vi "Driving.vi"(11 "Output Cluster in":T1) -> ()   [LabVIEW 2015]
uses:
  Joytsick/Controls to Cmmnds Output Clust.ctl
  Global Vars.vi
  <vilib>/Rock Robotics/WPI/Utilities/WPI_GetSetVariantRefNum.vi
  <vilib>/Rock Robotics/WPI/RobotDrive/WPI_RobotDriveMecanumDrive_Cartesian.vi
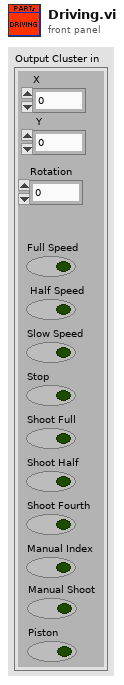
[diagram p1: front panel]
types:
  T1 = typedef "Controls to Cmmnds Output Clust.ctl" = cluster{"X ":dbl, " Y":dbl, "Rotation":dbl, "Full Speed":bool, " Half Speed":bool, "Slow Speed":bool, "Stop":bool, "Shoot Full":bool, "Shoot Half":bool, "Shoot Fourth":bool, "Manual Index":bool, "Piston":bool, "Manual Shoot":bool}
  T2 = typedef "WPI_RobotDriveDevRef.ctl" = cluster{"DevStatus":errorcluster, "Motors[]":T3[], "Square Inputs":bool, "Max Output":dbl}
  T3 = typedef "WPI_MotorControlDeviceRef.ctl" = cluster{"DeviceStatus":errorcluster, "Type":T4, "PWM":cluster{"PWM Channel":T5, "DeadBand":T6}, "CAN":cluster{"Device Number":u8, "Control Mode":T7, "Semaphore":T8, "Max Vout":dbl, "TalonSRX Control Mode":T9}, "Invert":bool}
  T4 = typedef "WPI_MotorControlType.ctl" = enum16{"PWM", "CAN", "CANTalonSRX"}
  T5 = typedef "FPGA_DIOPWMChannel.ctl" = enum8{"PWM 0", "PWM 1", "PWM 2", "PWM 3", "PWM 4", "PWM 5", "PWM 6", "PWM 7", "PWM 8", "PWM 9", "PWM MXP 0", "PWM MXP 1", "PWM MXP 2", "PWM MXP 3", "PWM MXP 4", "PWM MXP 5", "PWM MXP 6", "PWM MXP 7", "PWM MXP 8", "PWM MXP 9", "Invalid"}
  T6 = typedef "WPI_PWMDeadband.ctl" = cluster{"Name":string, "maxPositivePwm":i32, "minPositivePwm":i32, "centerPwm":i32, "maxNegativePwm":i32, "minNegativePwm":i32, "angularRange":u16}
  T7 = typedef "WPI_CANJaguar_ControlMode.ctl" = enum8{"Percent VBus", "Current", "Speed", "Position", "Voltage"}
  T8 = typedef "Semaphore RefNum" = refnum<k1>
  T9 = typedef "WPI_CANTalonSRX_APIControlMode.ctl" = enum8{"Percent VBus", "Speed", "Position", "Slave", "Unchanged / Invalid", "Voltage Compensation", "Current", "Motion Profile"}
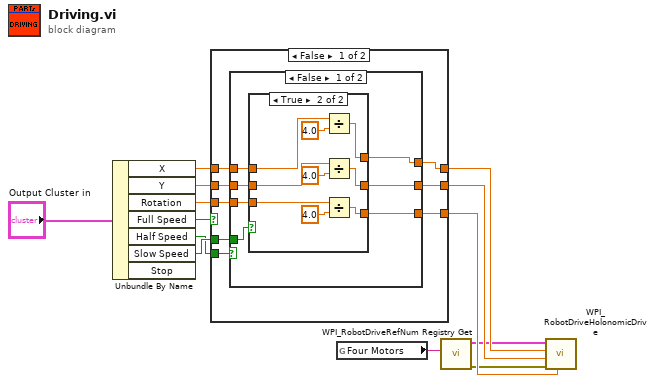
[diagram p0: block diagram]
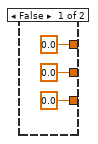
[diagram p2: hidden frame]
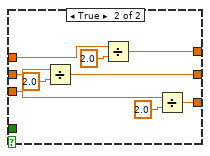
[diagram p3: hidden frame]
diagram:
  n1 = Unbundle By Name("Output Cluster in") -> ("X"=w7:dbl, "Y"=w8:dbl, "Rotation"=w10:dbl, "Full Speed"=w5:bool, "Half Speed"=w12:bool, "Slow Speed"=w13:bool)  [unwired: 1 out]
  n2 = case shown="False" w5 {
    tunnel: [w21 w52] -> w6
    tunnel: w7 -> [w20 w52]
    tunnel: [w19 w51] -> w9
    tunnel: w8 -> [w18 w51]
    tunnel: [w17 w50] -> w11
    tunnel: w10 -> [w16 w50]
    tunnel: w12 -> [w15 _]
    tunnel: w13 -> [w14 _]
    frame False {
      n3 = case shown="False" w15 {
        tunnel: [w22 w43] -> w21
        tunnel: w20 -> [w27 w49]
        tunnel: [w23 w42] -> w19
        tunnel: w18 -> [w26 w46]
        tunnel: [w24 w41] -> w17
        tunnel: w16 -> [w25 w47]
        tunnel: w14 -> [w28 _]
        frame False {
          n4 = case shown="True" w28 {
            tunnel: w27 -> [_ w37]
            tunnel: w26 -> [_ w36]
            tunnel: w25 -> [_ w35]
            tunnel: [0.0 w34] -> w24
            tunnel: [0.0 w33] -> w23
            tunnel: [0.0 w32] -> w22
            frame False {
            }
            frame True {
              n5 = Divide(x=w37, y=4.0) -> (x/y=w32:dbl)
              n6 = Divide(x=w36, y=4.0) -> (x/y=w33:dbl)
              n7 = Divide(x=w35, y=4.0) -> (x/y=w34:dbl)
            }
          }
        }
        frame True {
          n8 = Divide(x=w46, y=2.0) -> (x/y=w42:dbl)
          n9 = Divide(x=w49, y=2.0) -> (x/y=w43:dbl)
          n10 = Divide(x=w47, y=2.0) -> (x/y=w41:dbl)
        }
      }
    }
    frame True {
    }
  }
  n11 = global read "Global Vars.vi" "Four Motors"() -> (w1:string)
  n12 = call <vilib>:"WPI_RobotDriveRefNum Registry Get.vi"("refnum name"=w1) -> ("error out"=w3:errorcluster, "RobotDriveDevRef"=w2:T2)  [unwired: 9 in]
  n13 = call-poly <vilib>:"WPI_RobotDriveHolonomicDrive.vi"("Rotation"=w11, "error in (no error)"=w3, "Y"=w9, "X"=w6, "RobotDriveDevRef"=w2) -> ()  [unwired: 4 in, 3 out]
